vi "VCS Set Object_INT8.vi"(0 "axis In":cluster{"keyHandle":u32, "nodeId":u16}={"keyHandle"=0, "nodeId"=1}, 5 "object in":T1 {"object subIndex" format="%x"; "object index" format="%x"}, 11 "error in (no error)":errorcluster) -> (4 "axis Out":cluster{"keyHandle":u32, "nodeId":u16}={"keyHandle"=0, "nodeId"=1}, 15 "error out":errorcluster)   [LabVIEW 2017, in "maxonEPOS.lvlib"]
doc: "<B>VCS Set Object</B> writes an INT8 object value at the given index and sub index from object dictionary."
uses:
  Examples/maxonEPOS.lvlib
  SSI_Tool/InstrumentsInterfaces/Motordriver/maxon EPOS/Resources/EposCmd.dll
  SSI_Tool/InstrumentsInterfaces/Motordriver/maxon EPOS/Resources/EposCmd64.dll
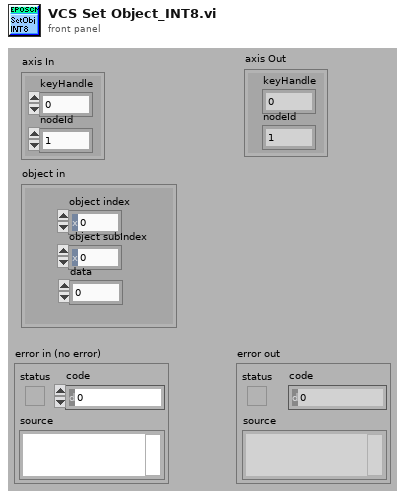
[diagram p1: front panel]
types:
  T1 = cluster{"object index":u16, "object subIndex":u8, "data":i8}
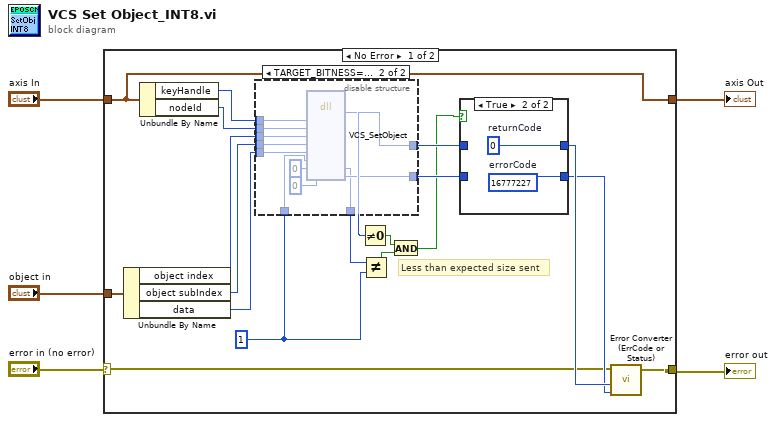
[diagram p0: block diagram]
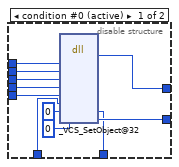
[diagram p2: hidden frame]
diagram:
  n1 = case shown="No Error" "error in (no error)" {
    selector: "error in (no error)" -> [w6 w51]
    tunnel: [w9 w51] -> w4
    tunnel: "axis In" -> [w12 w50]
    tunnel: "object in" -> [w23 _]
    tunnel: [w12 w50] -> w1
    frame No Error {
      w10 = u32 1
      # "Less than expected size sent"
      n2 = Unbundle By Name(w23) -> ("object index"=w20:u16, "object subIndex"=w19:u8, "data"=w11:i8)
      n3 = Unbundle By Name(w12) -> ("keyHandle"=w22:u32, "nodeId"=w21:u16)
      n4 = disable-structure shown="TARGET_BITNESS==64" {
        disable-tunnel: w22 -> [w34 w45]
        disable-tunnel: w21 -> [w33 w44]
        disable-tunnel: w20 -> [w32 w43]
        disable-tunnel: w19 -> [w31 w42]
        disable-tunnel: [w30 w41] -> w18
        disable-tunnel: [w29 w40] -> w17
        disable-tunnel: [w28 w39] -> w16
        disable-tunnel: w11 -> [w25 w36]
        disable-tunnel: w10 -> [w24 w35]
        frame condition #0 (active) {
          n5 = dll-call lib="C:/workspace/project/scancon/sw/SSI_Tool/InstrumentsInterfaces/Motordriver/maxon EPOS/Resources/EposCmd.*" fn="_VCS_SetObject@32"("KeyHandle"=w34, "NodeId"=w33, "ObjectIndex"=w32, "ObjectSubIndex"=w31, "Data"=w25, "NbOfBytesToWrite"=w24, "pNbOfBytesWritten"=u32 0, "pErrorCode"=u32 0) -> (w28:i32, "pNbOfBytesWritten"=w29:u32, "pErrorCode"=w30:u32)  [unwired: 9 in, 2 out]
        }
        frame condition #1 {
          n6 = dll-call lib="C:/setup/Resources/EposCmd64.*" fn="VCS_SetObject" ("EposCmd.dll:_VCS_SetObject@32")("KeyHandle"=w45, "NodeId"=w44, "ObjectIndex"=w43, "ObjectSubIndex"=w42, "Data"=w36, "NbOfBytesToWrite"=w35, "pNbOfBytesWritten"=u32 0, "pErrorCode"=u32 0) -> ("Rückgabetyp"=w39:i32, "pNbOfBytesWritten"=w40:u32, "pErrorCode"=w41:u32)  [unwired: 9 in, 2 out]
        }
      }
      n7 = Not Equal To 0?(x=w16) -> (x != 0?=w14:bool)
      n8 = Not Equal?(x=w17, y=w10) -> (x != y?=w15:bool)
      n9 = And(x=w14, y=w15) -> (x .and. y?=w13:bool)
      n10 = case shown="True" w13 {
        tunnel: [w47 w49] -> w8
        tunnel: [w46 w48] -> w7
        tunnel: w16 -> [w47 _]
        tunnel: w18 -> [w46 _]
        frame False {
        }
        frame True {
          w48 = u32 16777227  # errorCode
          w49 = 0  # returnCode
        }
      }
      n11 = call "Error Converter (ErrCode or Status).vi"("error code"=w7, "return type"=w8, "error in (no error)"=w6) -> ("error out"=w9:errorcluster)  [unwired: 7 in]
    }
    frame Error {
    }
  }
  "error out" <- w4
  "axis Out" <- w1
